vi "Map To Direction.vi"(11 "Theta":dbl) -> (2 "In Range?":bool, 3 "Direction":T1)   [LabVIEW 2011]
uses:
  Direction.ctl
panel:
  in  "Heading Data":cluster{"Heading":dbl, "Error":dbl}[](array[cluster])=[{"Heading"=0.0, "Error"=10.0}, {"Heading"=50.0, "Error"=12.0}, {"Heading"=90.0, "Error"=10.0}, {"Heading"=130.0, "Error"=12.0}, {"Heading"=180.0, "Error"=10.0}, {"Heading"=-130.0, "Error"=12.0}, {"Heading"=-90.0, "Error"=10.0}, {"Heading"=-50.0, "Error"=12.0}, {"Heading"=-180.0, "Error"=10.0}]
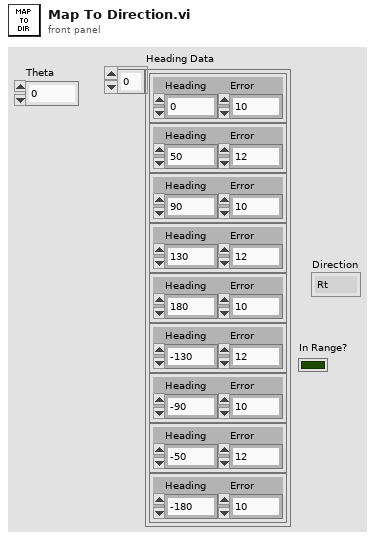
[diagram p1: front panel]
types:
  T1 = typedef "Direction.ctl" = enum16{"Rt", "Rt-Up", "Up", "Lt-Up", "Lt", "Lt-Dn", "Dn", "Rt-Dn", "Unknown"}
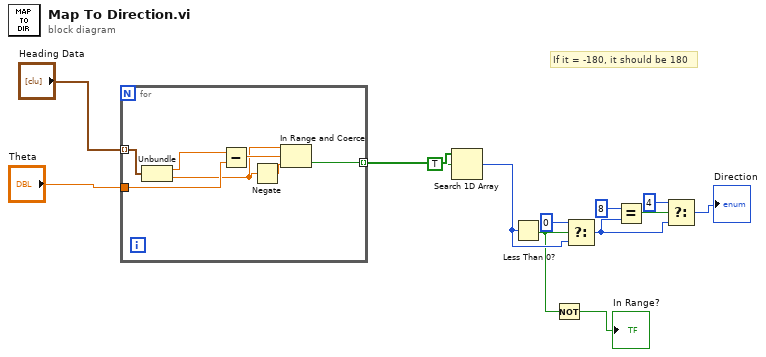
[diagram p0: block diagram]
diagram:
  # "If it = -180, it should be 180"
  n1 = for {
    tunnel: "Heading Data" -> [w20] mode=indexing
    tunnel: "Theta" -> [w18]
    tunnel: [w14] -> w11 mode=indexing
    n2 = Unbundle(w20) -> ("Heading"=w19:dbl, "Error"=w15:dbl)
    n3 = Subtract(x=w19, y=w18) -> (x-y=w17:dbl)
    n4 = Negate(x=w15) -> (-x=w16:dbl)
    n5 = In Range and Coerce(upper limit=w15, x=w17, lower limit=w16) -> (In Range?=w14:bool)  [unwired: 1 out]
  }
  n6 = Search 1D Array(1D array=w11, element=TRUE) -> (index of element=w9:i32)  [unwired: 1 in]
  n7 = Less Than 0?(x=w9) -> (x < 0?=w6:bool)
  n8 = Not(x=w6) -> (.not. x?=→"In Range?":bool)
  n9 = Select(t=0, s=w6, f=w9) -> (s? t:f=w3:i32)
  n10 = Equal?(x=8, y=w3) -> (x = y?=w4:bool)
  n11 = Select(t=4, s=w4, f=w3) -> (s? t:f=→"Direction":i32)
